vi "Highlight Plot.vi"(10 "PlotNum":i32, 11 "XYGraph in":refnum<vi>) -> ()   [LabVIEW 2015, in "Graph Extensions.lvlib"]
uses:
  Graph Extensions.lvlib
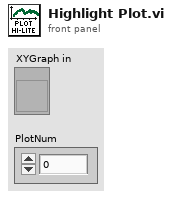
[diagram p1: front panel]
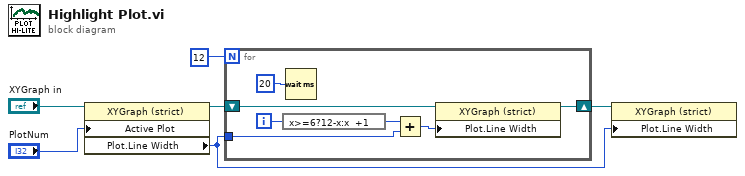
[diagram p0: block diagram]
diagram:
  n1 = property class="XYGraph (strict)"(reference="XYGraph in", "Active Plot"="PlotNum") -> (reference out=w2:refnum<vi>, "Plot.Line Width"=w5:u8)  [unwired: 1 in, 1 out]
  n2 = for {
    N: 12 -> [_]
    tunnel: w5 -> [w10]
    shift-right: [w12] -> w4
    shift-left: w2 -> [w13]
    i -> [w11]
    n3 = expression code="x>=6?12-x:x  +1"(w11) -> (w8:i32)
    n4 = Wait (ms)(milliseconds to wait=u32 20) -> ()  [unwired: 1 out]
    n5 = Add(x=w8, y=w10) -> (x+y=w9:i32)
    n6 = property class="XYGraph (strict)"(reference=w13, "Plot.Line Width"=w9) -> (reference out=w12:refnum<vi>)  [unwired: 1 in, 1 out]
  }
  n7 = property class="XYGraph (strict)"(reference=w4, "Plot.Line Width"=w5) -> ()  [unwired: 1 in, 2 out]
